vi "AO Out Only Engine.vi"(0 "Unique Notifier Name":string="Not a Name", 11 "AO Channel":string[](array[string])) -> ()   [LabVIEW 2020]
uses:
  External Power Control Type Defs/External Power Notifier Type.ctl
  External Power Control Type Defs/External Power Actions.ctl
  <vilib>/DAQmx/write.llb/DAQmx Write (Analog DBL 1Chan 1Samp).vi
  <vilib>/DAQmx/create/channels.llb/DAQmx Create Channel (AO-Voltage-Basic).vi
  <vilib>/DAQmx/miscellaneous.llb/DAQmx Fill In Error Info.vi
panel:
  in  "Power (%)":dbl
  in  "Quit":bool
  in  "Line On Off":bool
  # "Array Elements must be:\n\n1) AO Channel (e.g. Dev1/ao0)"
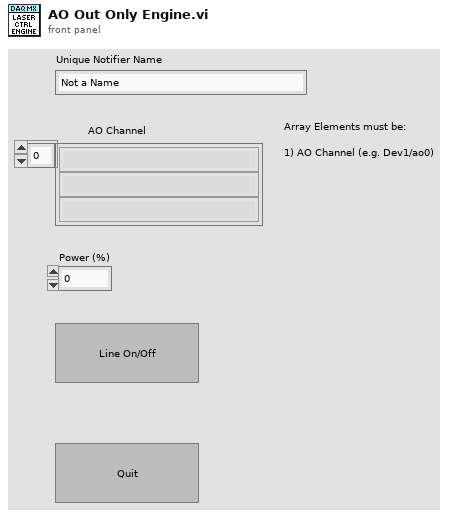
[diagram p1: front panel]
types:
  T1 = typedef "External Power Notifier Type.ctl" = cluster{"Actions":T2, "Wavelength":string, "Line On/Off":bool, "Power (%)":dbl, "Control Parameters":variant, "Cmd Done?":bool}
  T2 = typedef "External Power Actions.ctl" = enum16{"Line On/Off", "Set Power", "Set Ctrl Parameters", "Quit"}
  T3 = enum32{"Invalid", "Standard", "Closed", "Hidden", "Minimized", "Maximized"}
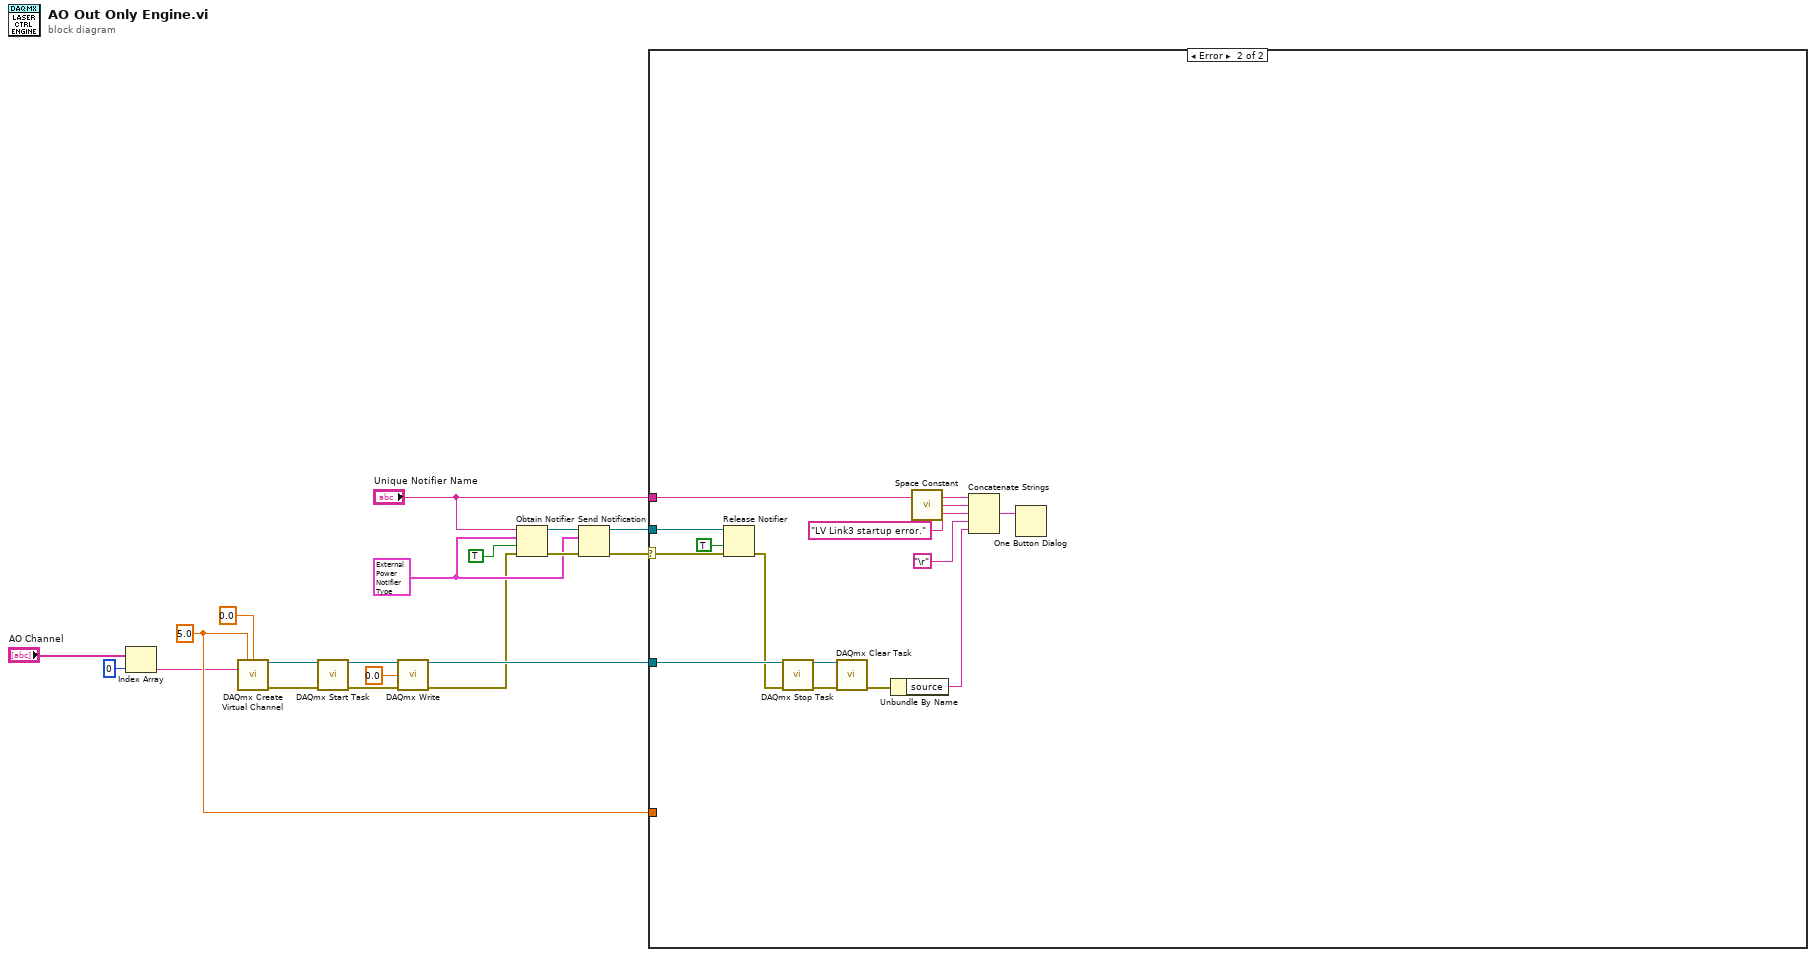
[diagram p0: block diagram]
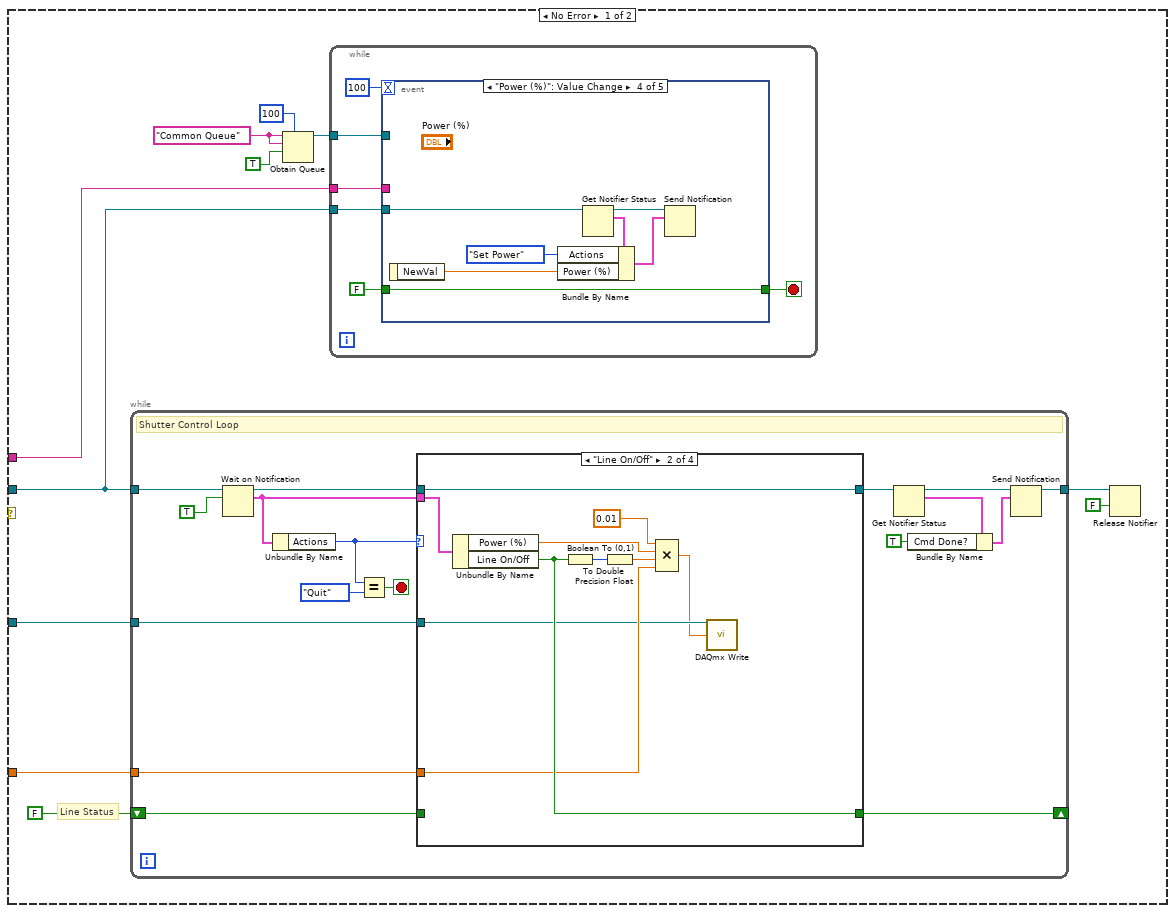
[diagram p2: hidden frame]
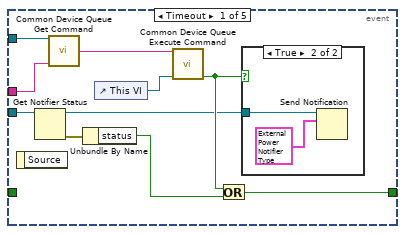
[diagram p3: hidden frame]
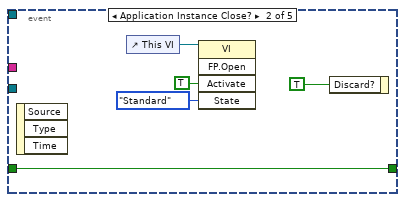
[diagram p5: hidden frame]
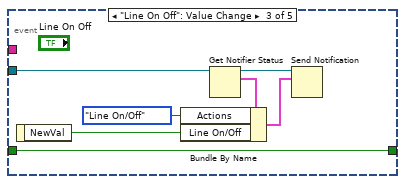
[diagram p6: hidden frame]
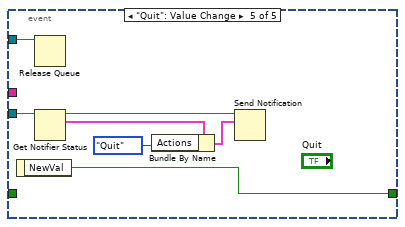
[diagram p7: hidden frame]
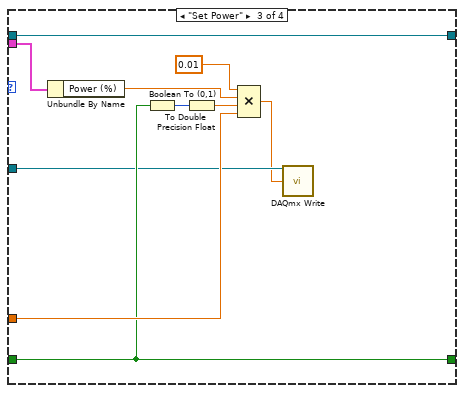
[diagram p9: hidden frame]
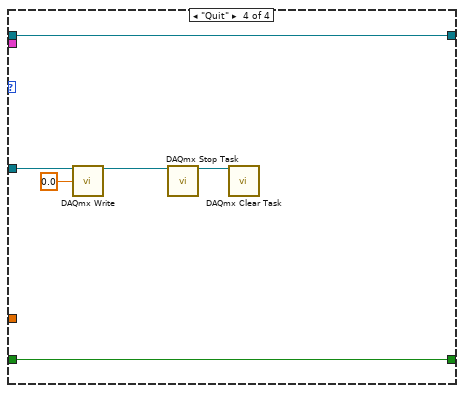
[diagram p10: hidden frame]
diagram:
  w10 = 5.0 ("maximum value")
  w15 = T1 {"Actions"=enum."Set Power", "Wavelength"="", "Line On/Off"=FALSE, "Power (%)"=0.0, "Control Parameters"=variant, "Cmd Done?"=FALSE} ("External Ctrl")
  n1 = Index Array(array="AO Channel", index=0) -> (element=w1:string)
  n2 = call-poly <vilib>:"DAQmx Create Virtual Channel.vi"("maximum value"=w10, "minimum value"=0.0, "physical channels"=w1) -> ("task out"=w6:refnum<k21>, "error out"=w5:errorcluster)  [unwired: 11 in]
  n3 = call <vilib>:"DAQmx Start Task.vi"("task/channels in"=w6, "error in"=w5) -> ("task out"=w4:refnum<k21>, "error out"=w3:errorcluster)  [unwired: 12 out]
  n4 = call-poly <vilib>:"DAQmx Write.vi"("task/channels in"=w4, "data"=0.0, "error in"=w3) -> ("task out"=w8:refnum<k21>, "error out"=w2:errorcluster)  [unwired: 10 in, 1 out]
  n5 = Obtain Notifier(name (unnamed)="Unique Notifier Name", notification data type=w15, create if not found? (T)=TRUE, error in (no error)=w2) -> (notifier out=w18:refnum<notifier>, error out=w17:errorcluster)  [unwired: 1 out]
  n6 = Send Notification(notification=w15, notifier=w18, error in (no error)=w17) -> (notifier out=w16:refnum<notifier>, error out=w14:errorcluster)
  n7 = case shown="Error" w14 {
    selector: w14 -> [_ w131]
    tunnel: w8 -> [w30 w122]
    tunnel: w16 -> [w28 w132]
    tunnel: "Unique Notifier Name" -> [w27 w130]
    tunnel: w10 -> [w21 _]
    frame No Error {
      w26 = "Common Queue" ("Unique Notifier Name")
      # "Line Status"
      n8 = while {
        tunnel: w28 -> [w83]
        tunnel: w30 -> [w89]
        tunnel: [w84] -> w20
        shift-right: [w76] -> _
        shift-left: FALSE -> [w77]
        tunnel: w21 -> [w75]
        stop <- w90 stop-if-true
        # "Shutter Control Loop"
        n9 = Wait on Notification(notifier=w83, ignore previous (F)=TRUE) -> (notifier out=w82:refnum<notifier>, notification=w81:T1)  [unwired: 2 in, 2 out]
        n10 = Unbundle By Name(w81) -> ("Actions"=w80:T2)
        n11 = Equal?(x=w80, y=External_Power_Actions."Quit") -> (x = y?=w90:bool)
        n12 = case shown="\"Line On/Off\"" w80 {
          tunnel: w82 -> [w93 w103 w113 w119]
          tunnel: w89 -> [_ w95 w105 w116]
          tunnel: [w93 w103 w113 w119] -> w87
          tunnel: w81 -> [_ w102 w112 _]
          tunnel: w77 -> [w92 _ w106 w118]
          tunnel: [w92 w100 w106 w118] -> w76
          tunnel: w75 -> [_ w96 w107 _]
          frame Default {
          }
          frame "Line On/Off" {
            n13 = Unbundle By Name(w102) -> ("Power (%)"=w98:dbl, "Line On/Off"=w100:bool)
            n14 = Boolean To (0,1)(Boolean=w100) -> (0, 1=w101:i16)
            n15 = To Double Precision Float(number=w101) -> (double precision float=w99:dbl)
            n16 = Compound Arithmetic op=MULTIPLY(0.01 ("value"), w98, w99, w96) -> (w94:dbl)
            n17 = call-poly <vilib>:"DAQmx Write.vi"("task/channels in"=w95, "data"=w94) -> ()  [unwired: 11 in, 3 out]
          }
          frame "Set Power" {
            n18 = Unbundle By Name(w112) -> ("Power (%)"=w109:dbl)
            n19 = Boolean To (0,1)(Boolean=w106) -> (0, 1=w111:i16)
            n20 = To Double Precision Float(number=w111) -> (double precision float=w110:dbl)
            n21 = Compound Arithmetic op=MULTIPLY(0.01 ("value"), w109, w110, w107) -> (w104:dbl)
            n22 = call-poly <vilib>:"DAQmx Write.vi"("task/channels in"=w105, "data"=w104) -> ()  [unwired: 11 in, 3 out]
          }
          frame "Quit" {
            n23 = call-poly <vilib>:"DAQmx Write.vi"("task/channels in"=w116, "data"=0.0) -> ("task out"=w114:refnum<k21>)  [unwired: 11 in, 2 out]
            n24 = call <vilib>:"DAQmx Stop Task.vi"("task/channels in"=w114) -> ("task out"=w115:refnum<k21>)  [unwired: 13 in, 1 out]
            n25 = call <vilib>:"DAQmx Clear Task.vi"("task in"=w115) -> ()  [unwired: 14 in, 1 out]
          }
        }
        n26 = Get Notifier Status(notifier=w87) -> (notifier out=w85:refnum<notifier>, current notification=w88:T1)  [unwired: 1 in, 3 out]
        n27 = Bundle By Name(cluster=w88, "Cmd Done?"=TRUE ("Received?")) -> (w78:T1)
        n28 = Send Notification(notification=w78, notifier=w85) -> (notifier out=w84:refnum<notifier>)  [unwired: 1 in, 1 out]
      }
      n29 = Obtain Queue(max queue size (-1, unlimited)=100, name (unnamed)=w26, element data type=w26, create if not found? (T)=TRUE) -> (queue out=w23:refnum<queue>)  [unwired: 1 in, 2 out]
      n30 = while {
        tunnel: w23 -> [w36]
        tunnel: w28 -> [w33]
        tunnel: w27 -> [w31]
        stop <- w32 stop-if-true
        n31 = event shown="[3] \"Power (%)\": Value Change" {
          selector: _ -> [_ _ _ _ _]
          dyn-events: _ -> [_ _ _ _ _]
          timeout: 100 -> [_ _ _ _ _]
          tunnel: w36 -> [w44 _ _ _ w69]
          tunnel: FALSE -> [_ w53 w56 w63 _]
          tunnel: w33 -> [w46 _ w60 w67 w70]
          tunnel: [w39 w53 w56 w63 w74] -> w32
          tunnel: w31 -> [w43 _ _ _ _]
          event Timeout {
            n32 = event-data() -> ()  [unwired: 1 in, 1 out]
            n33 = Get Notifier Status(notifier=w46) -> (notifier out=w37:refnum<notifier>, error out=w45:errorcluster)  [unwired: 1 in, 3 out]
            n34 = call "Common Device Queue Get Command.vi"("Common Queue"=w44, "Notifier Name"=w43) -> ("Command"=w42:string)  [unwired: 12 in, 1 out]
            n35 = Unbundle By Name(w45) -> ("status"=w40:bool)
            n36 = control-ref of="This VI"() -> (w41:refnum<vi>)
            n37 = call "Common Device Queue Execute Command.vi"("Common Command"=w42, "VI Refnum"=w41) -> ("Quit?"=w38:bool)  [unwired: 12 in, 1 out]
            n38 = Or(x=w38, y=w40) -> (x .or. y?=w39:bool)
            n39 = case shown="True" w38 {
              tunnel: w37 -> [_ w48]
              frame False {
              }
              frame True {
                n40 = Send Notification(notification=T1 {"Actions"=enum."Quit", "Wavelength"="", "Line On/Off"=FALSE, "Power (%)"=0.0, "Control Parameters"=variant, "Cmd Done?"=FALSE} ("External Ctrl"), notifier=w48) -> ()  [unwired: 1 in, 2 out]
              }
            }
          }
          event Application Instance Close? {
            n41 = event-data() -> ()  [unwired: 1 in, 3 out]
            n42 = control-ref of="This VI"() -> (w50:refnum<vi>)
            n43 = invoke class="VI" method="FP.Open"(reference=w50, "Activate"=TRUE ("Activate?"), "State"=T3."Standard") -> ()  [unwired: 2 in, 5 out]
            n44 = event-data("Discard?"=TRUE) -> ()  [unwired: 1 in, 1 out]
          }
          event "Line On Off": Value Change {
            n45 = event-data() -> ("NewVal"=w55:bool)  [unwired: 1 in]
            n46 = Get Notifier Status(notifier=w60) -> (notifier out=w59:refnum<notifier>, current notification=w58:T1)  [unwired: 1 in, 3 out]
            n47 = Bundle By Name(cluster=w58, "Actions"=External_Power_Actions."Line On/Off", "Line On/Off"=w55) -> (w57:T1)
            n48 = Send Notification(notification=w57, notifier=w59) -> ()  [unwired: 1 in, 2 out]
          }
          event "Power (%)": Value Change {
            n49 = event-data() -> ("NewVal"=w62:dbl)  [unwired: 1 in]
            n50 = Get Notifier Status(notifier=w67) -> (notifier out=w66:refnum<notifier>, current notification=w65:T1)  [unwired: 1 in, 3 out]
            n51 = Bundle By Name(cluster=w65, "Actions"=External_Power_Actions."Set Power", "Power (%)"=w62) -> (w64:T1)
            n52 = Send Notification(notification=w64, notifier=w66) -> ()  [unwired: 1 in, 2 out]
          }
          event "Quit": Value Change {
            n53 = event-data() -> ("NewVal"=w74:bool)  [unwired: 1 in]
            n54 = Release Queue(queue=w69) -> ()  [unwired: 2 in, 3 out]
            n55 = Get Notifier Status(notifier=w70) -> (notifier out=w73:refnum<notifier>, current notification=w72:T1)  [unwired: 1 in, 3 out]
            n56 = Bundle By Name(cluster=w72, "Actions"=External_Power_Actions."Quit") -> (w71:T1)
            n57 = Send Notification(notification=w71, notifier=w73) -> ()  [unwired: 1 in, 2 out]
          }
        }
      }
      n58 = Release Notifier(notifier=w20, force destroy? (F)=FALSE) -> ()  [unwired: 1 in, 3 out]
    }
    frame Error {
      n59 = Release Notifier(notifier=w132, force destroy? (F)=TRUE, error in (no error)=w131) -> (error out=w121:errorcluster)  [unwired: 2 out]
      n60 = call <vilib>:"DAQmx Stop Task.vi"("task/channels in"=w122, "error in"=w121) -> ("task out"=w124:refnum<k21>, "error out"=w123:errorcluster)  [unwired: 12 in]
      n61 = call <vilib>:"DAQmx Clear Task.vi"("task in"=w124, "error in"=w123) -> ("error out"=w120:errorcluster)  [unwired: 13 out]
      n62 = Unbundle By Name(w120) -> ("source"=w125:string)
      n63 = call <vilib>:"Space Constant.vi"() -> ("String"=w128:string)
      n64 = Concatenate Strings(w130, w128, "LV Link3 startup error." ("string"), "\r", w125) -> (w129:string)
      n65 = One Button Dialog(message=w129) -> ()  [unwired: 1 in, 1 out]
    }
  }
